vi "fit-function_v03__with_pars_and_eval_node_v02.vi"(9 "coefficients":dbl[](array[numeric])=[12.849354442227447, 5.866421178332907, 12.080788064739096, 5.80910915007397, 1224.8335576996235, 9.529730177350924] format="%.6f", 10 "x":dbl[](array[numeric]), 11 "formula":string) -> (2 "parameter":string[](array[string]), 3 "y":dbl[](graph))   [LabVIEW 2010]
panel:
  out "error out":errorcluster
  in  "error in":errorcluster
  out "function\nvariables":string[](array[string])
  # "Needs:\na funtion in C syntax with variables a0, a1, a2, ...\ncoefficients for the variables\nx values\n\nReturns:\ny values\n\n\nif the number of coefficients supplied don't\nmatch the number of variables in the formula,\nthe array of coefficients will be pruned or fulled\nup with  0's."
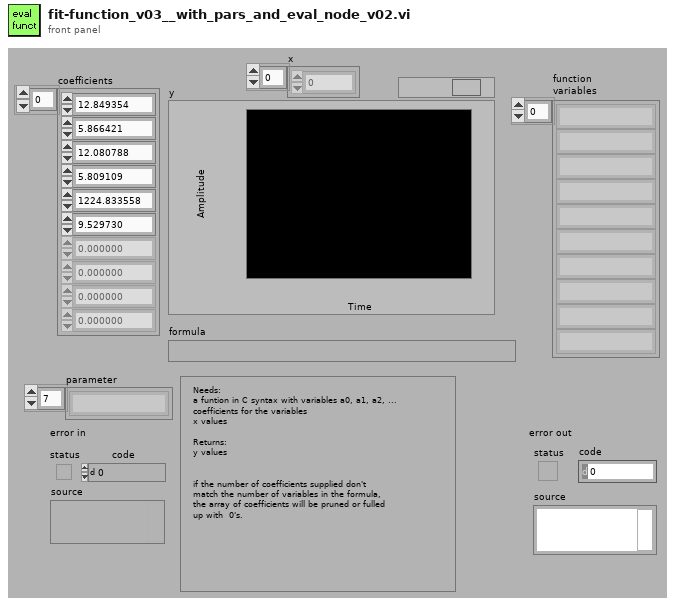
[diagram p1: front panel]
types:
  T1 = cluster{"Y Values":dbl[][], "Tables":i32[][][], "Variables input decode":i32[], "Variables output decode":i32[]}
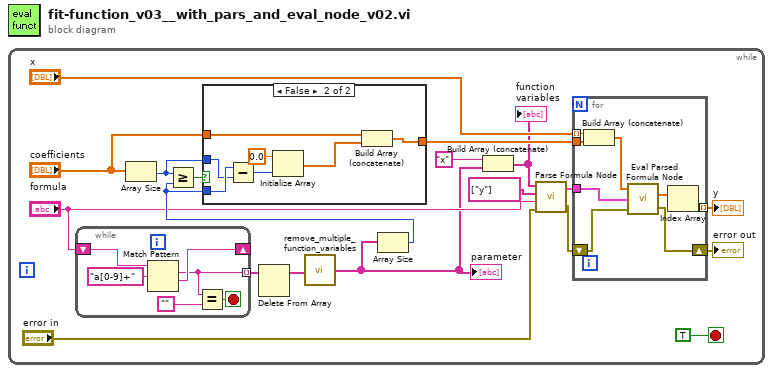
[diagram p0: block diagram]
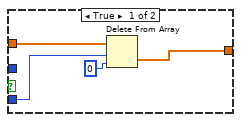
[diagram p2: hidden frame]
diagram:
  n1 = while {
    stop <- TRUE stop-if-true
    n2 = while {
      tunnel: [w41] -> w18 mode=indexing
      shift-right: [w42] -> _
      shift-left: "formula" -> [w44]
      stop <- w39 stop-if-true
      n3 = Match Pattern(string=w44, regular expression="a[0-9]+") -> (match substring=w41:string, after substring=w42:string)  [unwired: 1 in, 2 out]
      n4 = Equal?(x=w41, y="") -> (x = y?=w39:bool)
    }
    n5 = Array Size(array="coefficients") -> (size(s)=w11:i32)
    n6 = Delete From Array(array=w18) -> (array with subset deleted=w2:string[])  [unwired: 2 in, 1 out]
    n7 = call "remove_multiple_function_variables.vi"("function\nvariables"=w2) -> ("unique\nfunction\nvariables"=w1:string[])
    "parameter" <- w1
    n8 = Array Size(array=w1) -> (size(s)=w12:i32)
    n9 = Greater Or Equal?(x=w11, y=w12) -> (x >= y?=w13:bool)
    n10 = case shown="False" w13 {
      tunnel: "coefficients" -> [w23 w29]
      tunnel: [w21 w30] -> w14
      tunnel: w12 -> [w22 w28]
      tunnel: w11 -> [_ w27]
      frame True {
        n11 = Delete From Array(array=w23, length=w22, index=0) -> (deleted portion=w21:dbl[])  [unwired: 1 out]
      }
      frame False {
        n12 = Subtract(x=w28, y=w27) -> (x-y=w26:i32)
        n13 = Initialize Array(0.0 ("element"), w26) -> (w24:dbl[])
        n14 = Build Array (concatenate)(w29, w24) -> (w30:dbl[])
      }
    }
    n15 = Build Array (concatenate)("x" ("formula"), w1) -> (w9:string[])
    "function\nvariables" <- w9
    n16 = call "Parse Formula Node.vi"("error in (no error)"="error in", "formula"="formula", "Variables Output"=string[] ["y"], "Variables Input"=w9) -> ("error out"=w4:errorcluster, "Parsed Formula Node"=w5:T1)
    n17 = for {
      tunnel: w14 -> [w37]
      tunnel: "x" -> [w38] mode=indexing
      tunnel: [w34] -> w17 mode=indexing
      tunnel: w5 -> [w33]
      shift-right: [w32] -> w3
      shift-left: w4 -> [w31]
      n18 = Build Array (concatenate)(w38, w37) -> (w36:dbl[])
      n19 = call "Eval Parsed Formula Node.vi"("error in (no error)"=w31, "Parsed Formula Node"=w33, "Input Values"=w36) -> ("error out"=w32:errorcluster, "Output Values"=w35:dbl[])
      n20 = Index Array(array=w35) -> (element=w34:dbl)  [unwired: 1 in]
    }
    "y" <- w17
    "error out" <- w3
  }
